vi "ParseArguments.vi"(8 "error in (no error)":errorcluster, 9 "Inputs":string[](array[string]), 11 "UniquifyFullyQualifiedVIName in":refnum<class "UniquifyFullyQualifiedVIName.lvclass">) -> (0 "error out":errorcluster, 3 "UniquifyFullyQualifiedVIName out":refnum<class "UniquifyFullyQualifiedVIName.lvclass">)   [LabVIEW 2015, in "UniquifyFullyQualifiedVIName.lvclass"]
uses:
  UniquifyFullyQualifiedVIName.lvclass
  UniquifyFullyQualifiedVIName.lvclass/UniquifyFullyQualifiedVIName.ctl
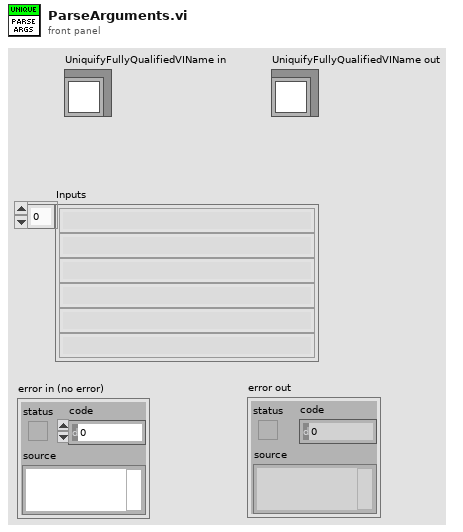
[diagram p1: front panel]
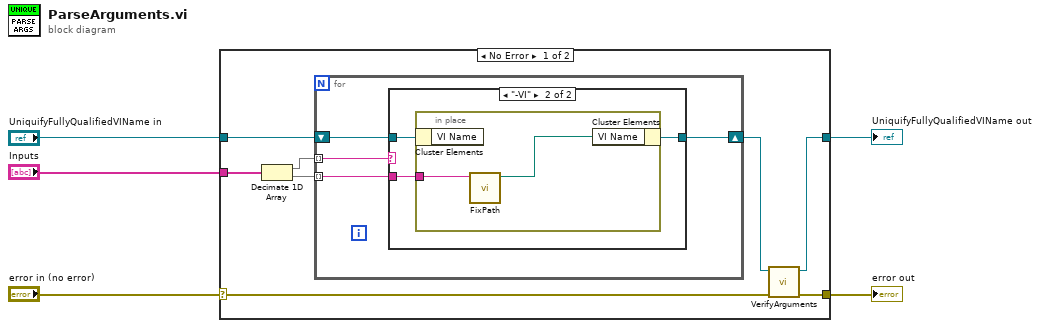
[diagram p0: block diagram]
diagram:
  n1 = case shown="No Error" "error in (no error)" {
    selector: "error in (no error)" -> [w8 w25]
    tunnel: [w9 w25] -> w4
    tunnel: "UniquifyFullyQualifiedVIName in" -> [w11 w24]
    tunnel: "Inputs" -> [w10 _]
    tunnel: [w6 w24] -> w1
    frame No Error {
      n2 = Decimate 1D Array(w10) -> (w12:string[], w13:string[])
      n3 = for {
        tunnel: w12 -> [w17] mode=indexing
        tunnel: w13 -> [w15] mode=indexing
        shift-right: [w14] -> w7
        shift-left: w11 -> [w16]
        n4 = case shown="\"-VI\"" w17 {
          tunnel: w16 -> [w18 w21]
          tunnel: w15 -> [_ w20]
          tunnel: [w18 w19] -> w14
          frame Default {
          }
          frame "-VI" {
            n5 = in-place {
              in-place-border: w20 -> [w23]
              n6 = in-place-cluster #1(w21) -> ()  [unwired: 1 out]
              n7 = call "FixPath.vi"("path string"=w23) -> ("path"=w22:path)  [unwired: 10 in]
              n8 = in-place-cluster #1("VI Name"=w22) -> (w19:refnum<class "UniquifyFullyQualifiedVIName.lvclass">)
            }
          }
        }
      }
      n9 = call "VerifyArguments.vi"("error in (no error)"=w8, "UniquifyFullyQualifiedVIName in"=w7) -> ("error out"=w9:errorcluster, "UniquifyFullyQualifiedVIName out"=w6:refnum<class "UniquifyFullyQualifiedVIName.lvclass">)  [unwired: 8 in]
    }
    frame Error {
    }
  }
  "error out" <- w4
  "UniquifyFullyQualifiedVIName out" <- w1
